vi "All SubFunctions 4.vi"(4 "מק\"ט המכלל":string, 5 "מספר סידורי":string, 7 "מפעיל":string="ANS", 8 "error":errorcluster, 11 "Path for Log":path) -> (0 "error IO":errorcluster)   [LabVIEW 2014]
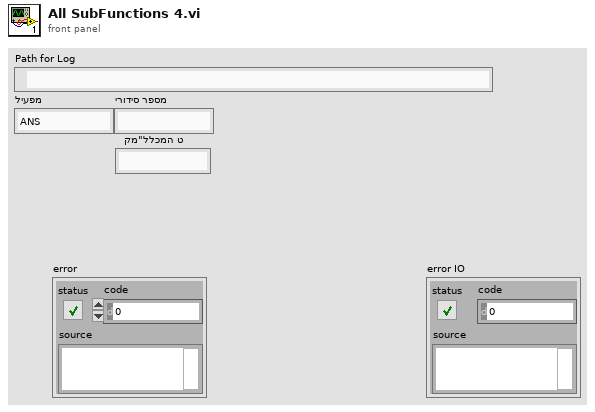
[diagram p1: front panel]
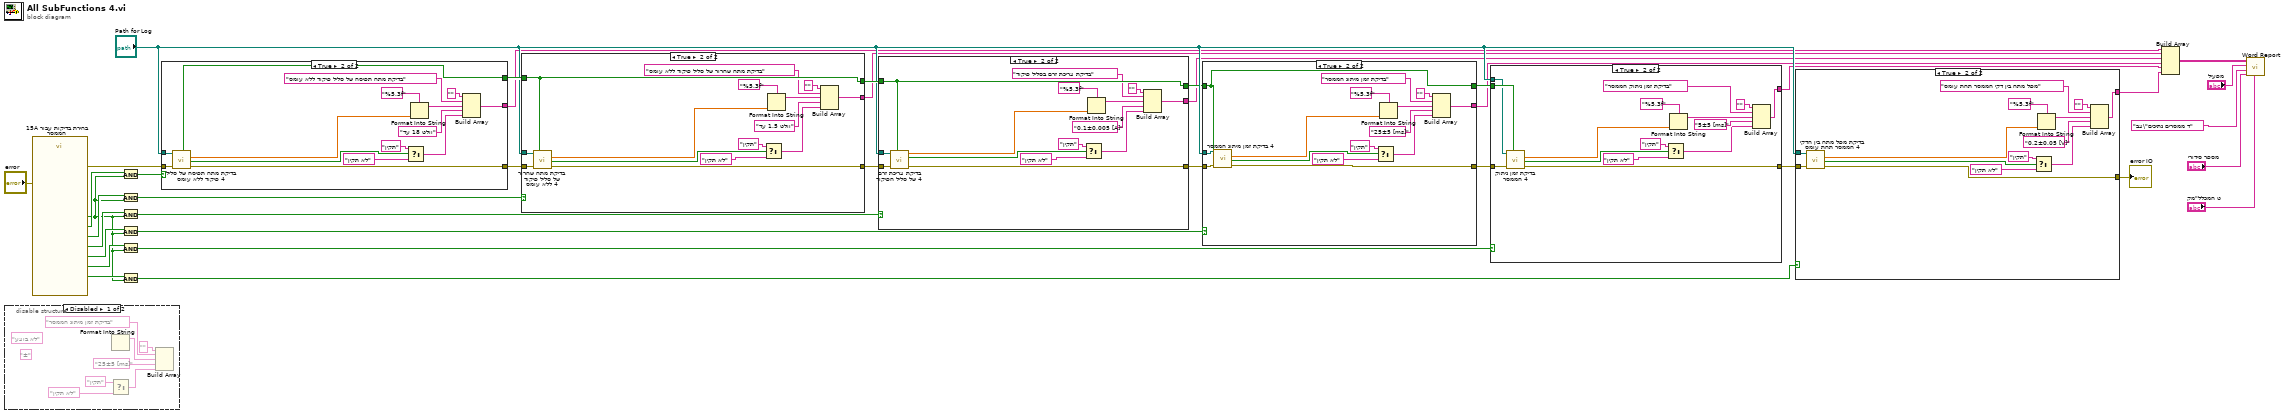
[diagram p0: block diagram]
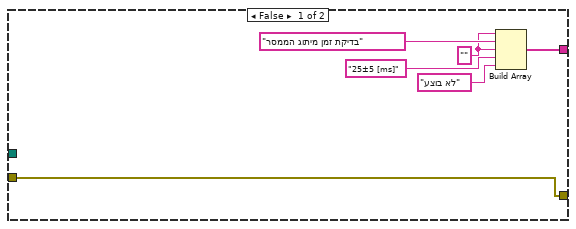
[diagram p3: hidden frame]
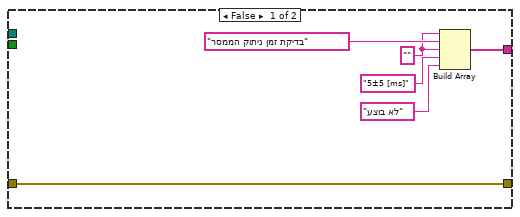
[diagram p4: hidden frame]
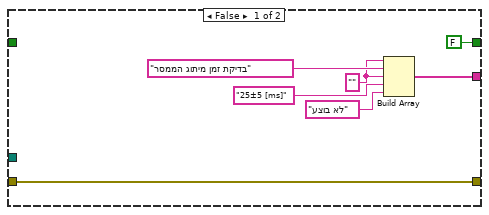
[diagram p5: hidden frame]
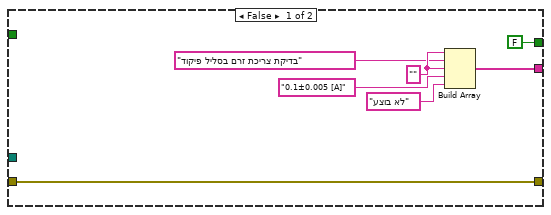
[diagram p6: hidden frame]
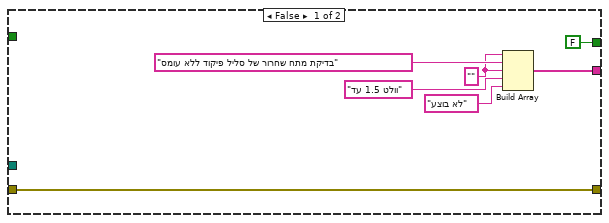
[diagram p7: hidden frame]
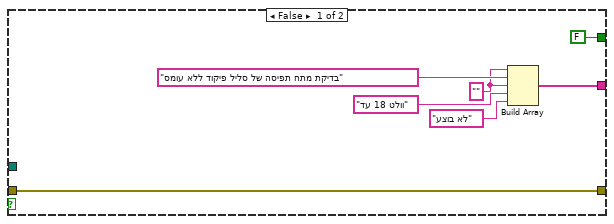
[diagram p8: hidden frame]
diagram:
  n1 = disable-structure shown="Disabled" {
    frame Disabled {
      (unwired) "±"
      (unwired) "לא בוצע"
      n2 = Format Into String() -> (resulting string=w42:string)  [unwired: 4 in, 1 out]
      n3 = Select(t="תקין", f="לא תקין") -> (s? t:f=w44:string)  [unwired: 1 in]
      n4 = Build Array("" ("element"), "בדיקת זמן מיתוג הממסר" ("element"), w42, "25±5 [ms]" ("element"), w44) -> ()  [unwired: 1 out]
    }
    frame Enabled {
    }
  }
  n5 = call "15A בחירת בדיקות עבור הממסר.vi"("error in (no error)"="error") -> ("בדיקת מפל מתח בין דקי הממסר תחת עומס"=w20:bool, "בדיקת זמן ניתוק הממסר"=w22:bool, "בדיקת זמן מיתוג הממסר"=w24:bool, "בדיקת צריכת זרם של סליל הפיקוד"=w26:bool, "בדיקת מתח שחרור של סליל פיקוד ללא עומס"=w28:bool, "בדיקת מתח תפיסה של סליל פיקוד ללא עומס"=w18:bool, "OK"=w17:bool, "error out"=w30:errorcluster)  [unwired: 10 in, 1 out]
  n6 = And(x=w18, y=w17) -> (x .and. y?=w29:bool)
  n7 = And(x=w28, y=w17) -> (x .and. y?=w27:bool)
  n8 = And(x=w26, y=w17) -> (x .and. y?=w25:bool)
  n9 = And(x=w24, y=w17) -> (x .and. y?=w23:bool)
  n10 = And(x=w22, y=w17) -> (x .and. y?=w21:bool)
  n11 = And(x=w20, y=w17) -> (x .and. y?=w19:bool)
  n12 = case shown="True" w29 {
    tunnel: [w51 w66] -> w32
    tunnel: w30 -> [w51 w65]
    tunnel: "Path for Log" -> [_ w64]
    tunnel: [FALSE ("resultUserPrompt") w63] -> w16
    tunnel: [w47 w53] -> w11
    frame False {
      w46 = "" ("element")
      n13 = Build Array(w46, "בדיקת מתח תפיסה של סליל פיקוד ללא עומס" ("element"), w46, "עד 18 וולט" ("element"), "לא בוצע") -> (w47:string[])
    }
    frame True {
      n14 = call "בדיקת מתח תפיסה של סליל פיקוד ללא עומס 4.vi"("error"=w65, "Path for Log"=w64) -> ("error out"=w66:errorcluster, "מצב ממסר פתוח/סגור"=w60:bool, "מתח סגירת הממסר"=w59:dbl, "resultUserPrompt"=w63:bool)  [unwired: 5 in, 1 out]
      n15 = Select(t="תקין", s=w60, f="לא תקין") -> (s? t:f=w54:string)
      n16 = Format Into String(format string="%5.3f", w59) -> (resulting string=w55:string)  [unwired: 2 in, 1 out]
      n17 = Build Array("" ("element"), "בדיקת מתח תפיסה של סליל פיקוד ללא עומס" ("element"), w55, "עד 18 וולט" ("element"), w54) -> (w53:string[])
    }
  }
  n18 = case shown="True" w27 {
    tunnel: w32 -> [w73 w88]
    tunnel: [w73 w87] -> w31
    tunnel: "Path for Log" -> [_ w86]
    tunnel: w16 -> [_ w85]
    tunnel: [FALSE ("resultUserPrompt") w85] -> w15
    tunnel: [w67 w75] -> w9
    frame False {
      w68 = "" ("element")
      n19 = Build Array(w68, "בדיקת מתח שחרור של סליל פיקוד ללא עומס" ("element"), w68, "עד 1.5 וולט" ("element"), "לא בוצע") -> (w67:string[])
    }
    frame True {
      n20 = call "בדיקת מתח שחרור של סליל פיקוד ללא עומס 4.vi"("resultUserPrompt"=w85, "error"=w88, "Path for Log"=w86) -> ("error out"=w87:errorcluster, "מצב ממסר פתוח/סגור"=w81:bool, "מתח פתיחת הממסר"=w82:dbl)  [unwired: 5 in, 1 out]
      n21 = Select(t="תקין", s=w81, f="לא תקין") -> (s? t:f=w76:string)
      n22 = Format Into String(format string="%5.3f", w82) -> (resulting string=w78:string)  [unwired: 2 in, 1 out]
      n23 = Build Array("" ("element"), "בדיקת מתח שחרור של סליל פיקוד ללא עומס" ("element"), w78, "עד 1.5 וולט" ("element"), w76) -> (w75:string[])
    }
  }
  n24 = case shown="True" w25 {
    tunnel: [w95 w110] -> w35
    tunnel: w31 -> [w95 w109]
    tunnel: "Path for Log" -> [_ w108]
    tunnel: w15 -> [_ w107]
    tunnel: [FALSE ("resultUserPrompt") w107] -> w13
    tunnel: [w89 w97] -> w8
    frame False {
      w93 = "" ("element")
      n25 = Build Array(w93, "בדיקת צריכת זרם בסליל פיקוד" ("element"), w93, "0.1±0.005 [A]" ("element"), "לא בוצע") -> (w89:string[])
    }
    frame True {
      n26 = call "בדיקת צריכת זרם של סליל הפיקוד 4.vi"("resultUserPrompt"=w107, "error"=w109, "Path for Log"=w108) -> ("error out"=w110:errorcluster, "צריכת זרם בסליל בטווח כן/לא"=w100:bool, "צריכת זרם בסליל"=w101:dbl)  [unwired: 6 in]
      n27 = Select(t="תקין", s=w100, f="לא תקין") -> (s? t:f=w99:string)
      n28 = Format Into String(format string="%5.3f", w101) -> (resulting string=w98:string)  [unwired: 2 in, 1 out]
      n29 = Build Array("" ("element"), "בדיקת צריכת זרם בסליל פיקוד" ("element"), w98, "0.1±0.005 [A]" ("element"), w99) -> (w97:string[])
    }
  }
  n30 = case shown="True" w23 {
    tunnel: w35 -> [w117 w132]
    tunnel: [w117 w131] -> w34
    tunnel: "Path for Log" -> [_ w130]
    tunnel: w13 -> [_ w118]
    tunnel: [FALSE ("resultUserPrompt") w118] -> w12
    tunnel: [w111 w120] -> w7
    frame False {
      w113 = "" ("element")
      n31 = Build Array(w113, "בדיקת זמן מיתוג הממסר" ("element"), w113, "25±5 [ms]" ("element"), "לא בוצע") -> (w111:string[])
    }
    frame True {
      n32 = call "בדיקת זמן מיתוג הממסר 4.vi"("resultUserPrompt"=w118, "error"=w132, "Path for Log"=w130) -> ("error out"=w131:errorcluster, "בטוח כן/לא"=w122:bool, "בדיקת זמן מיתוג הממסר"=w121:dbl)  [unwired: 6 in]
      n33 = Select(t="תקין", s=w122, f="לא תקין") -> (s? t:f=w123:string)
      n34 = Format Into String(format string="%5.3f", w121) -> (resulting string=w125:string)  [unwired: 2 in, 1 out]
      n35 = Build Array("" ("element"), "בדיקת זמן מיתוג הממסר" ("element"), w125, "25±5 [ms]" ("element"), w123) -> (w120:string[])
    }
  }
  n36 = case shown="True" w21 {
    tunnel: w34 -> [w138 w153]
    tunnel: [w138 w152] -> w33
    tunnel: "Path for Log" -> [_ w139]
    tunnel: w12 -> [_ w151]
    tunnel: [w133 w141] -> w6
    frame False {
      w134 = "" ("element")
      n37 = Build Array(w134, "בדיקת זמן ניתוק הממסר" ("element"), w134, "5±5 [ms]" ("element"), "לא בוצע") -> (w133:string[])
    }
    frame True {
      n38 = call "בדיקת זמן ניתוק הממסר 4.vi"("resultUserPrompt"=w151, "error"=w153, "Path for Log"=w139) -> ("error out"=w152:errorcluster, "בטוח כן/לא"=w142:bool, "בדיקת זמן ניתוק הממסר"=w143:dbl)  [unwired: 6 in]
      n39 = Select(t="תקין", s=w142, f="לא תקין") -> (s? t:f=w144:string)
      n40 = Format Into String(format string="%5.3f", w143) -> (resulting string=w146:string)  [unwired: 2 in, 1 out]
      n41 = Build Array("" ("element"), "בדיקת זמן ניתוק הממסר" ("element"), w146, "5±5 [ms]" ("element"), w144) -> (w141:string[])
    }
  }
  n42 = case shown="True" w19 {
    tunnel: [w159 w173] -> w36
    tunnel: w33 -> [w159 w172]
    tunnel: "Path for Log" -> [_ w171]
    tunnel: [w154 w161] -> w5
    frame False {
      w155 = "" ("element")
      n43 = Build Array(w155, "בדיקת זמן מיתוג הממסר" ("element"), w155, "25±5 [ms]" ("element"), "לא בוצע") -> (w154:string[])
    }
    frame True {
      n44 = call "בדיקת מפל מתח בין הדקי הממסר תחת עומס 4.vi"("error"=w172, "Path for Log"=w171) -> ("error IO"=w173:errorcluster, "בטווח כן/לא"=w162:bool, "מפל מתח בין דקי הממסר תחת עומס"=w163:dbl)  [unwired: 6 in, 1 out]
      n45 = Select(t="תקין", s=w162, f="לא תקין") -> (s? t:f=w164:string)
      n46 = Format Into String(format string="%5.3f", w163) -> (resulting string=w166:string)  [unwired: 2 in, 1 out]
      n47 = Build Array("" ("element"), "מפל מתח בין דקי הממסר תחת עומס" ("element"), w166, "0.2±0.05 [V]" ("element"), w164) -> (w161:string[])
    }
  }
  "error IO" <- w36
  n48 = Build Array(w11, w9, w8, w7, w6, w5) -> (w10:string[][])
  n49 = call "Word Report.vi"("מק\"ט המכלל"="מק\"ט המכלל", "מספר סידורי"="מספר סידורי", "שם הצב\"ד"="צב\"ד ממסרים נתיכים", "מפעיל"="מפעיל", "Array"=w10) -> ()  [unwired: 7 in]
